vi "CameraIonView.vi"(10 "bound cluster in":T1, 11 "large camera view":dbl[][](array[numeric])) -> (2 "fluo counts":dbl, 3 "ion cam view":dbl[][](array[numeric]))   [LabVIEW 2017]
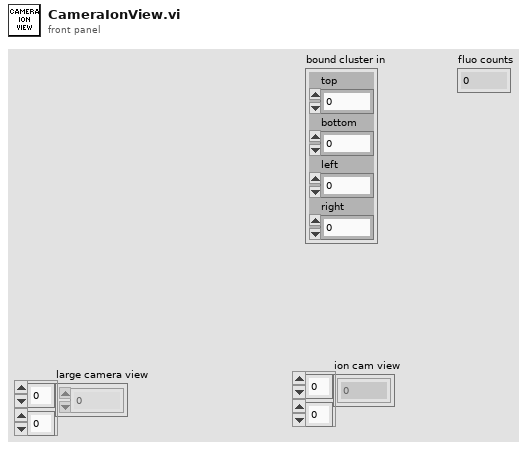
[diagram p1: front panel]
types:
  T1 = cluster{"top":i16, "bottom":i16, "left":i16, "right":i16}
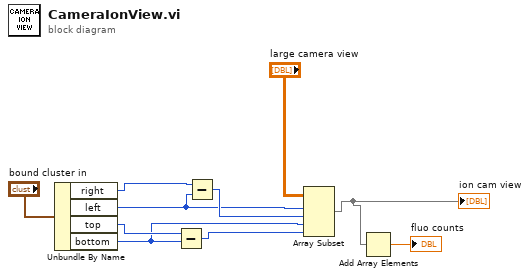
[diagram p0: block diagram]
diagram:
  n1 = Unbundle By Name("bound cluster in") -> ("right"=w8:i16, "left"=w6:i16, "top"=w5:i16, "bottom"=w3:i16)
  n2 = Subtract(x=w5, y=w3) -> (x-y=w4:i16)
  n3 = Subtract(x=w8, y=w6) -> (x-y=w7:i16)
  n4 = Array Subset(array="large camera view", index (row)=w6, length (row)=w7, index (col)=w3, length (col)=w4) -> (w2:dbl[][])
  "ion cam view" <- w2
  n5 = Add Array Elements(numeric array=w2) -> (sum=→"fluo counts":dbl)
